vi "Motion planning.vi"(0 "Command":dbl, 1 "Root length":dbl, 2 "Section length":dbl, 3 "Times":i32, 4 "Set":bool) -> (5 "Result":dbl[][](array[numeric]))   [LabVIEW 2018]
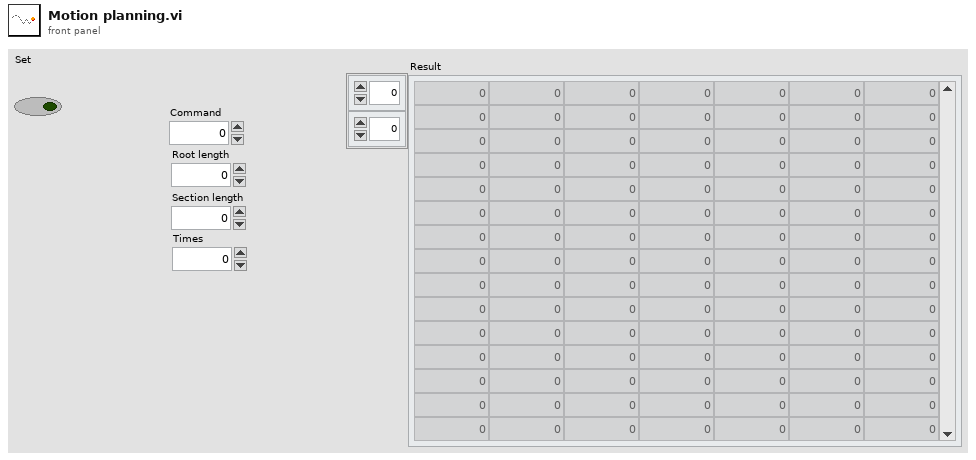
[diagram p1: front panel]
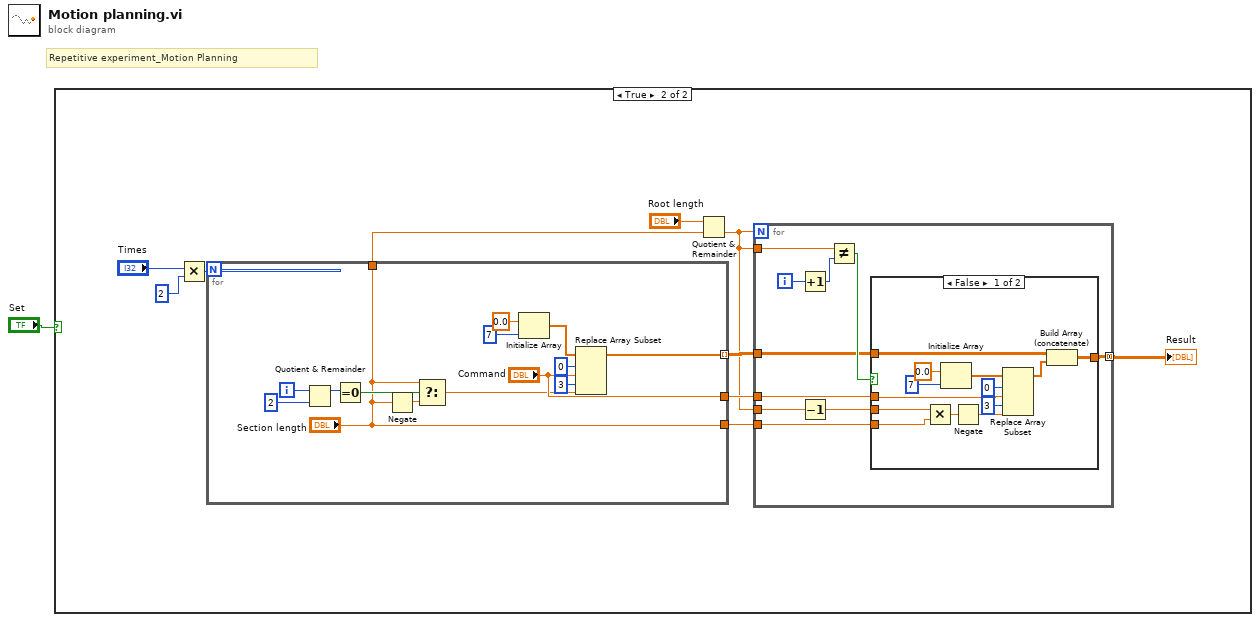
[diagram p0: block diagram]
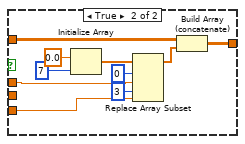
[diagram p3: hidden frame]
diagram:
  # "Repetitive experiment_Motion Planning"
  n1 = case shown="True" "Set" {
    frame False {
    }
    frame True {
      n2 = Multiply(x="Times", y=2) -> (x*y=w11:i32)
      n3 = for {
        N: w11 -> [_]
        tunnel: [w19] -> w7 mode=indexing
        tunnel: ["Command"] -> w8
        tunnel: ["Section length"] -> w3
        tunnel: ["Section length"] -> w2
        i -> [w18]
        n4 = Quotient & Remainder(x=w18, y=2) -> (x-y*floor(x/y)=w16:i32)  [unwired: 1 out]
        n5 = Equal To 0?(x=w16) -> (x = 0?=w15:bool)
        n6 = Negate(x="Section length") -> (-x=w13:dbl)
        n7 = Select(t="Section length", s=w15, f=w13) -> (s? t:f=w12:dbl)
        n8 = Initialize Array(0.0 ("element"), 7 ("dimension size")) -> (w23:dbl[])
        n9 = Replace Array Subset(array=w23, new element #1="Command", index #1=0 ("index"), new element #2=w12, index #2=3 ("index")) -> (w19:dbl[])
      }
      n10 = Quotient & Remainder(x="Root length", y=w2) -> (floor(x/y)=w4:dbl)  [unwired: 1 out]
      n11 = for {
        N: w4 -> [_]
        tunnel: w7 -> [w32]
        tunnel: w8 -> [w34]
        tunnel: w3 -> [w33]
        tunnel: [w31] -> w5 mode=concatenating
        tunnel: w4 -> [w30]
        tunnel: w4 -> [w27]
        i -> [w29]
        n12 = Increment(x=w29) -> (x+1=w28:i32)
        n13 = Decrement(x=w27) -> (x-1=w26:dbl)
        n14 = Not Equal?(x=w30, y=w28) -> (x != y?=w35:bool)
        n15 = case shown="False" w35 {
          tunnel: w34 -> [w42 w52]
          tunnel: w33 -> [w39 w51]
          tunnel: w32 -> [w41 w50]
          tunnel: [w43 w49] -> w31
          tunnel: w26 -> [w38 _]
          frame False {
            n16 = Multiply(x=w38, y=w39) -> (x*y=w37:dbl)
            n17 = Initialize Array(0.0 ("element"), 7 ("dimension size")) -> (w46:dbl[])
            n18 = Negate(x=w37) -> (-x=w36:dbl)
            n19 = Replace Array Subset(array=w46, new element #1=w42, index #1=0 ("index"), new element #2=w36, index #2=3 ("index")) -> (w44:dbl[])
            n20 = Build Array (concatenate)(w41, w44) -> (w43:dbl[][])
          }
          frame True {
            n21 = Initialize Array(0.0 ("element"), 7 ("dimension size")) -> (w56:dbl[])
            n22 = Replace Array Subset(array=w56, new element #1=w52, index #1=0 ("index"), new element #2=w51, index #2=3 ("index")) -> (w53:dbl[])
            n23 = Build Array (concatenate)(w50, w53) -> (w49:dbl[][])
          }
        }
      }
      "Result" <- w5
    }
  }
